vi "Download_Latest_Centauro_MC_Build_Skynet.vi"(0 "Save Path":path=path "C:/Automation/cibuilds/Centauro", 11 "Error In":errorcluster) -> (4 "Cent MC Path":path, 8 "Build Version":string, 15 "Error Out":errorcluster)   [LabVIEW 2016]
uses:
  <vilib>/regexp/Match Regular Expression.xnode
  <vilib>/httpClient/LabVIEWHTTPClient.lvlib
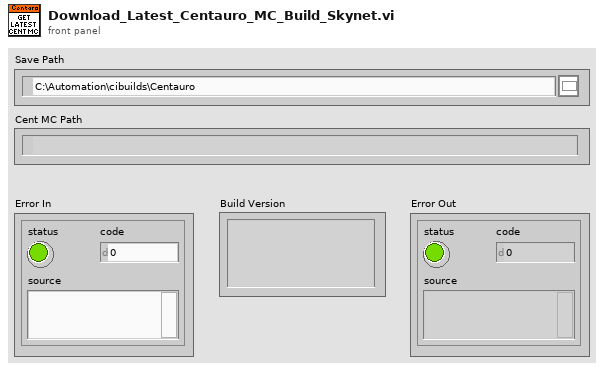
[diagram p1: front panel]
types:
  T1 = typedef "LabVIEWHTTPClient.lvlib/ClientHandle.ctl" = refnum<k1>
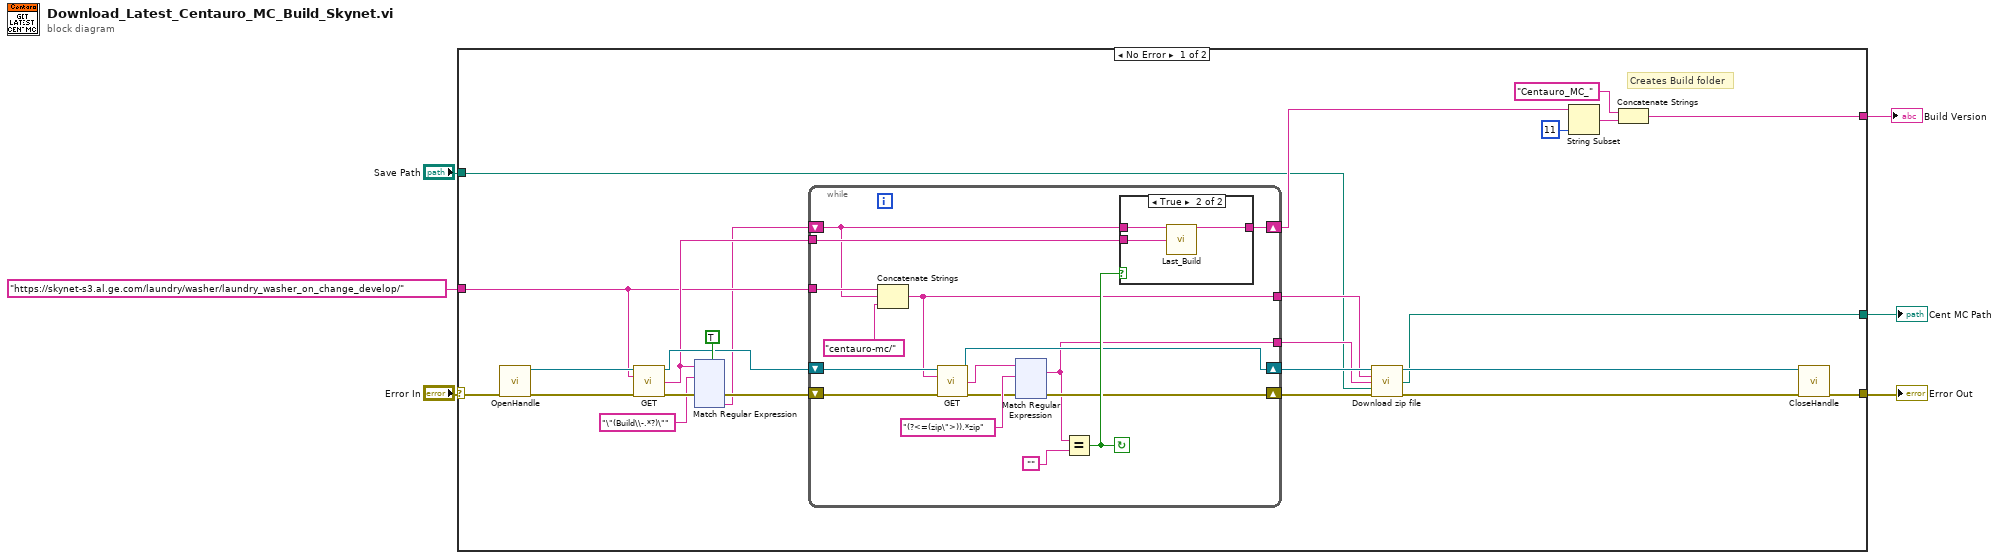
[diagram p0: block diagram]
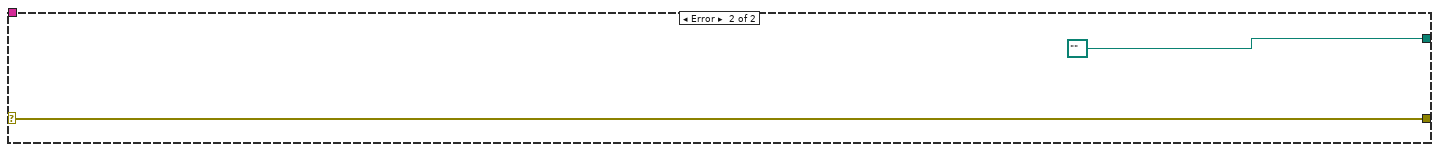
[diagram p3: hidden frame]
diagram:
  n1 = case shown="No Error" "Error In" {
    selector: "Error In" -> [w31 w283]
    tunnel: "https://skynet-s3.al.ge.com/laundry/washer/laundry_washer_on_change_develop/" -> [w21 _]
    tunnel: [w25 w283] -> w4
    tunnel: "Save Path" -> [w9 _]
    tunnel: [w7 path "" ("Output Path")] -> w2
    tunnel: [w16 _] -> w1
    frame No Error {
      # "Creates Build folder"
      n2 = call <vilib>:"OpenHandle.vi"("error in (no error)"=w31) -> ("client handle out"=w29:T1, "error out"=w30:errorcluster)  [unwired: 13 in]
      n3 = call <vilib>:"GET.vi"("client handle"=w29, "url"=w21, "error in (no error)"=w30) -> ("client handle out"=w23:T1, "body"=w22:string, "error out"=w28:errorcluster)  [unwired: 9 in, 1 out]
      n4 = xnode "Match Regular Expression"("input string"=w22, "regular expression"="\"(Build\\-.*?)\"", "error in"=w28, "multiline? (F)"=TRUE) -> ("error out"=w24:errorcluster, "submatch 1"=w8:string)  [unwired: 2 in, 4 out]
      n5 = while {
        shift-right: [w34] -> w15
        shift-left: w24 -> [w46]
        shift-right: [w35] -> w12
        shift-left: w23 -> [w45]
        tunnel: [w32] -> w11
        tunnel: w22 -> [w43]
        shift-right: [w42] -> w19
        shift-left: w8 -> [w40]
        tunnel: w21 -> [w41]
        tunnel: [w39] -> w10
        stop <- w44 continue-if-true
        n6 = Concatenate Strings(w41, w40, "centauro-mc/") -> (w39:string)
        n7 = call <vilib>:"GET.vi"("client handle"=w45, "url"=w39, "error in (no error)"=w46) -> ("client handle out"=w35:T1, "body"=w33:string, "error out"=w36:errorcluster)  [unwired: 9 in, 1 out]
        n8 = xnode "Match Regular Expression"("input string"=w33, "regular expression"="(?<=(zip\">)).*zip", "error in"=w36) -> ("whole match"=w32:string, "error out"=w34:errorcluster)  [unwired: 3 in, 3 out]
        n9 = Equal?(x=w32, y="") -> (x = y?=w44:bool)
        n10 = case shown="True" w44 {
          tunnel: w43 -> [_ w165]
          tunnel: w40 -> [w162 w164]
          tunnel: [w162 w163] -> w42
          frame False {
          }
          frame True {
            n11 = call "Last_Build.vi"("Current Build"=w164, "Webpage Source"=w165) -> ("Next Build"=w163:string)  [unwired: 13 in]
          }
        }
      }
      n12 = call "Download zip file.vi"("client handle"=w12, "Artifactory ZIP Directory"=w10, "Zip File"=w11, "Save Path"=w9, "Error In"=w15) -> ("client handle out"=w13:T1, "Output Path"=w7:path, "Error Out"=w14:errorcluster)  [unwired: 7 in, 1 out]
      n13 = String Subset(string=w19, length (rest)=11 ("length (rest)")) -> (substring=w18:string)  [unwired: 1 in]
      n14 = Concatenate Strings("Centauro_MC_" ("string"), w18) -> (w16:string)
      n15 = call <vilib>:"CloseHandle.vi"("client handle"=w13, "error in (no error)"=w14) -> ("error out"=w25:errorcluster)  [unwired: 13 in]
    }
    frame Error {
    }
  }
  "Error Out" <- w4
  "Cent MC Path" <- w2
  "Build Version" <- w1
